vi "Get Server gRPC UEs.vi"(11 "OOP Server in":refnum<class "Template Server.lvclass">) -> (2 "Server gRPC UEs":T1, 3 "OOP Server out":refnum<class "Template Server.lvclass">)   [LabVIEW 2019, in "Template Server.lvlib" / "Template Server.lvclass"]
uses:
  Template Server.lvclass
  typeDefs/Server gRPC UEs.ctl
  gRPC lvSupport/Server API/typeDefs/grpcId.ctl
  gRPC lvSupport/gprc-lvsupport.lvlib
  gRPC lvSupport/Server API/typeDefs/gRPCId Cluster.ctl
  gRPC lvSupport/Server API/typeDefs/gRPCId Cluster UE.ctl
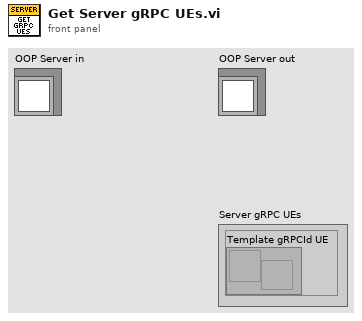
[diagram p1: front panel]
types:
  T1 = typedef "Template Server.lvlib/Template Server.lvclass/Server gRPC UEs.ctl" = cluster{"Template gRPCId UE":T2}
  T2 = typedef "Template Server.lvlib/gprc-lvsupport.lvlib/gRPCId Cluster UE.ctl" = refnum<user-event>
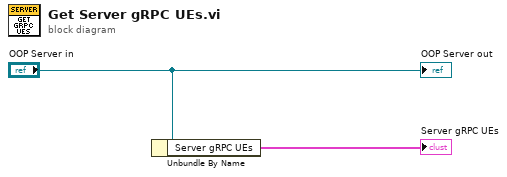
[diagram p0: block diagram]
diagram:
  n1 = Unbundle By Name("OOP Server in") -> ("Server gRPC UEs"=→"Server gRPC UEs":T1)
  "OOP Server out" <- "OOP Server in"
